vi "TDMS - Perform Group Props 2D.vi"(8 "error in (no error)":errorcluster, 10 "1D STR Array":string[](array[string]), 11 "2D STR Array in":string[][](array[string])) -> (0 "error out":errorcluster, 3 "2D STR Array out":string[][](array[string]))   [LabVIEW 2017]
doc: "This SubVI get channels names (1D), add last record as TimeStamp\nand past it as last column (description) into 2D array of other group properties."
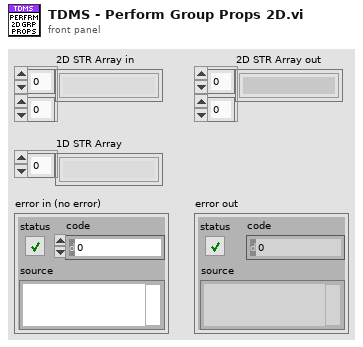
[diagram p1: front panel]
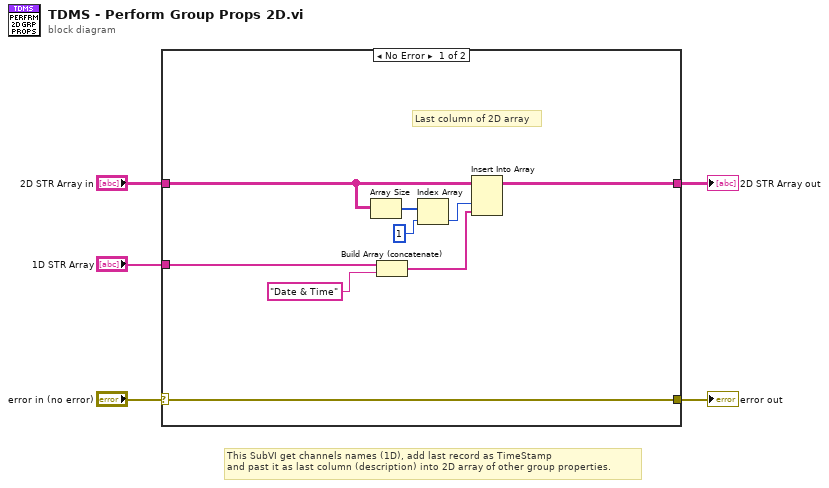
[diagram p0: block diagram]
diagram:
  # "This SubVI get channels names (1D), add last record as TimeStamp\nand past it as last column (description) into 2D array of other group properties."
  n1 = case shown="No Error" "error in (no error)" {
    selector: "error in (no error)" -> [w14 w15]
    tunnel: [w14 w15] -> w4
    tunnel: "2D STR Array in" -> [w10 _]
    tunnel: "1D STR Array" -> [w9 _]
    tunnel: [w6 _] -> w1
    frame No Error {
      # "Last column of 2D array"
      n2 = Array Size(array=w10) -> (size(s)=w13:i32[])
      n3 = Build Array (concatenate)(w9, "Date & Time") -> (w7:string[])
      n4 = Index Array(array=w13, index=1) -> (element=w11:i32)
      n5 = Insert Into Array(array=w10, index (col)=w11, new element=w7) -> (w6:string[][])  [unwired: 1 in]
    }
    frame Error {
    }
  }
  "error out" <- w4
  "2D STR Array out" <- w1
